vi "ArrayOfClustersWithStrings.vi"(11 "Array":T2(array[cluster])) -> (3 "Array 2":T1(array[cluster]))   [LabVIEW 2012]
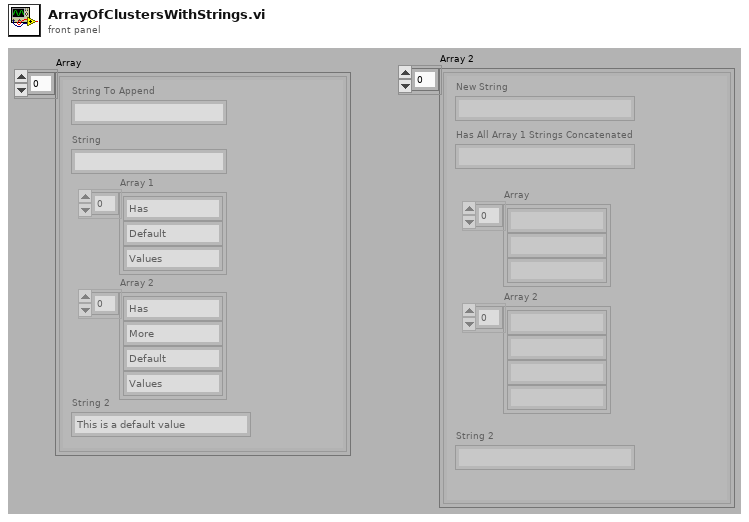
[diagram p1: front panel]
types:
  T1 = cluster{"New String":string, "Has All Array 1 Strings Concatenated":string, "Array":string[], "Array 2":string[], "String 2":string}[]
  T2 = cluster{"String To Append":string, "String":string, "Array 1":string[], "Array 2":string[], "String 2":string}[]
  T3 = cluster{"New String":string, "Has All Array 1 Strings Concatenated":string, "Array":string[], "Array 2":string[], "String 2":string}
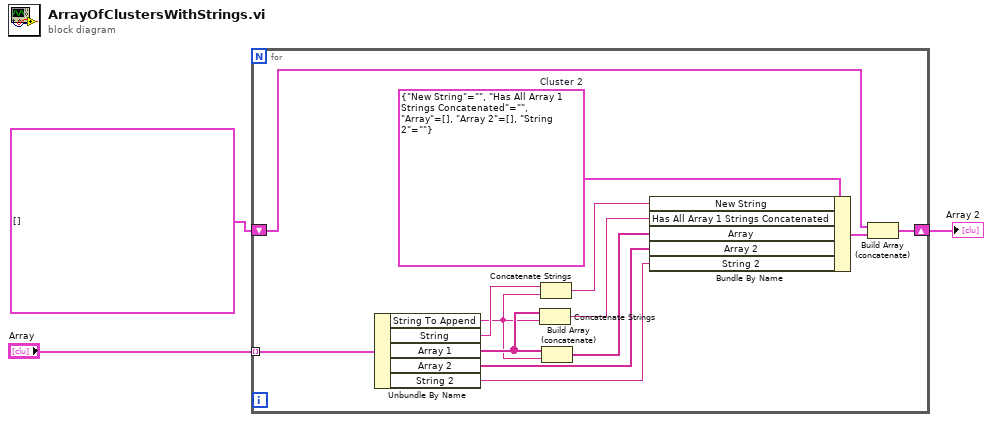
[diagram p0: block diagram]
diagram:
  n1 = for {
    tunnel: "Array" -> [w16] mode=indexing
    shift-right: [w13] -> w1
    shift-left: T1 [] -> [w15]
    w12 = T3 {"New String"="", "Has All Array 1 Strings Concatenated"="", "Array"=[], "Array 2"=[], "String 2"=""}  # Cluster 2
    n2 = Unbundle By Name(w16) -> ("String To Append"=w4:string, "String"=w11:string, "Array 1"=w6:string[], "Array 2"=w8:string[], "String 2"=w7:string)
    n3 = Concatenate Strings(w6, w4) -> (w9:string)
    n4 = Concatenate Strings(w11, w4) -> (w10:string)
    n5 = Build Array (concatenate)(w6, w4) -> (w5:string[])
    n6 = Bundle By Name(cluster=w12, "New String"=w10, "Has All Array 1 Strings Concatenated"=w9, "Array"=w5, "Array 2"=w8, "String 2"=w7) -> (w14:T3)
    n7 = Build Array (concatenate)(w15, w14) -> (w13:T1)
  }
  "Array 2" <- w1
